vi "Handle Command.vi"(8 "error in (no error)":errorcluster, 9 "Data":variant, 10 "Command":string, 11 "Inst.Xeryon-Rotator in":refnum<class "Inst.Xeryon-Rotator.lvclass">) -> (0 "error out":errorcluster, 1 "Processed Data":variant, 2 "Command":string, 3 "Inst.Xeryon-Rotator out":refnum<class "Inst.Xeryon-Rotator.lvclass">)   [LabVIEW 2019, in "Inst.Xeryon-Rotator.lvclass"]
uses:
  Inst.Xeryon-Rotator.lvclass
  Inst.Xeryon-Rotator.lvclass/Inst.Xeryon-Rotator.ctl
  <userlib>/LevyLab/Instrument Framework/Instrument Types/Cryostat/Instrument.Cryostat.lvclass
  <userlib>/LevyLab/Instrument Framework/Instrument Types/Cryostat/Typedefs/getAngle--cluster.ctl
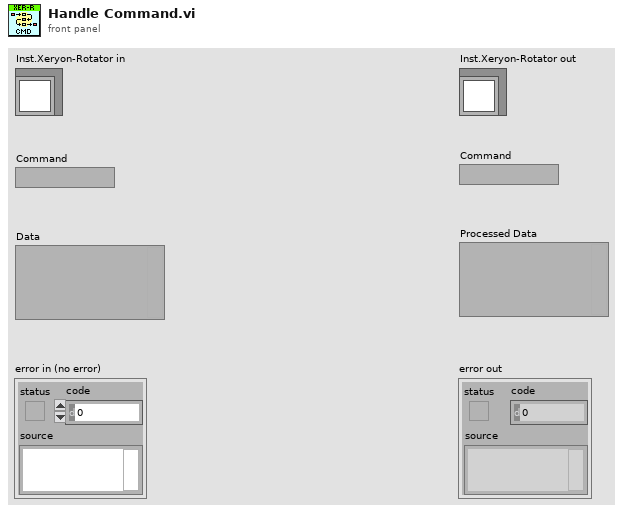
[diagram p1: front panel]
types:
  T1 = typedef "Instrument.Cryostat.lvclass/getAngle--cluster.ctl" = cluster{"angle":dbl, "status":string, "finished":bool}
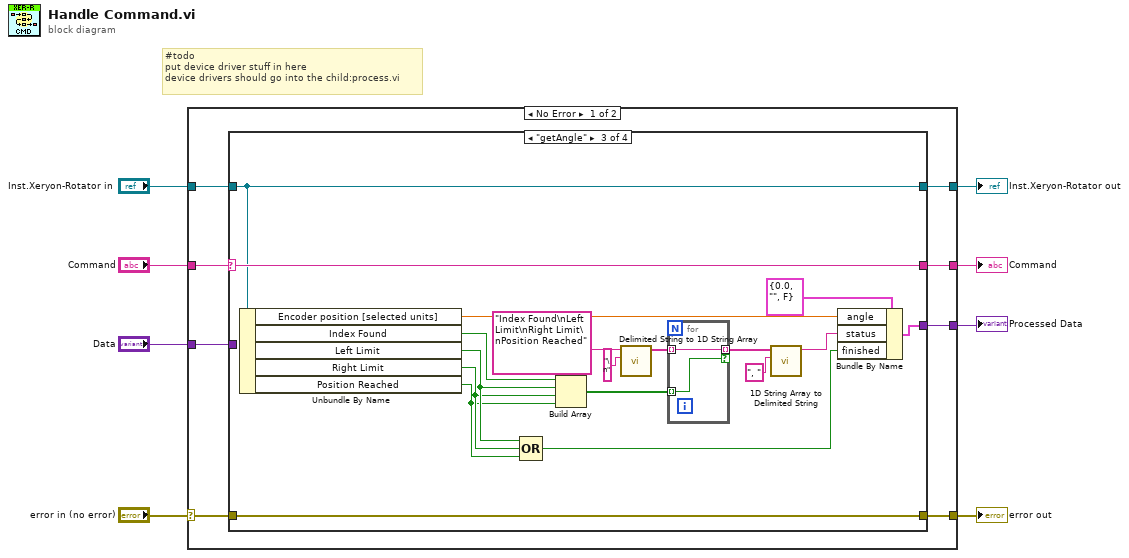
[diagram p0: block diagram]
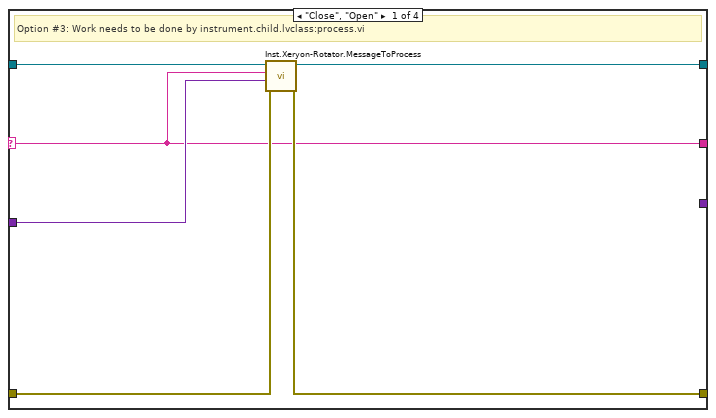
[diagram p2: hidden frame]
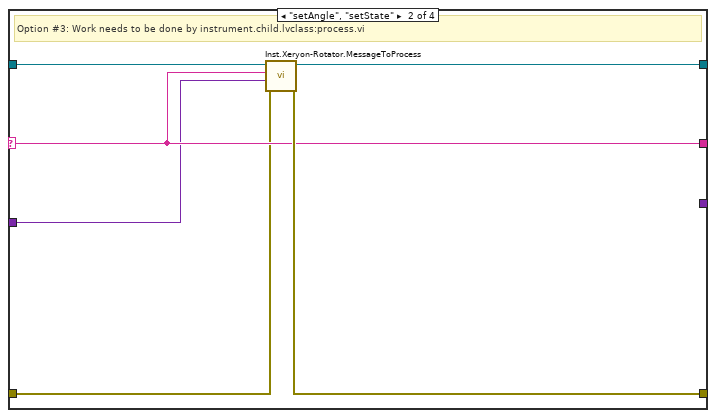
[diagram p3: hidden frame]
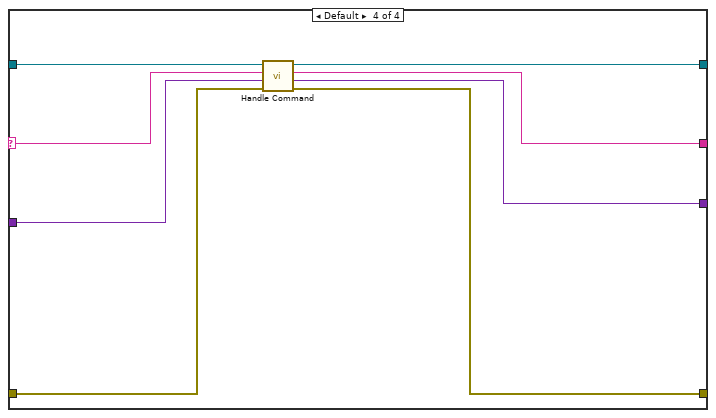
[diagram p4: hidden frame]
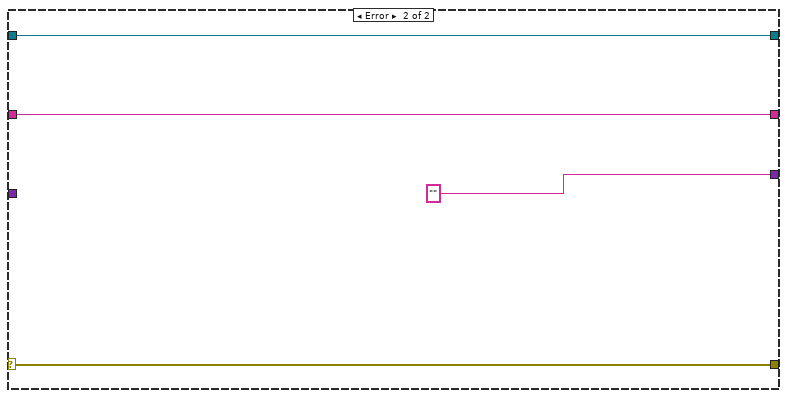
[diagram p5: hidden frame]
diagram:
  # "#todo\nput device driver stuff in here\ndevice drivers should go into the child:process.vi"
  n1 = case shown="No Error" "error in (no error)" {
    selector: "error in (no error)" -> [w10 w60]
    tunnel: [w12 w60] -> w6
    tunnel: [w14 w59] -> w5
    tunnel: "Inst.Xeryon-Rotator in" -> [w15 w59]
    tunnel: "Command" -> [w16 w57]
    tunnel: [w13 "" ("String")] -> w3
    tunnel: "Data" -> [w9 _]
    tunnel: [w11 w57] -> w1
    frame No Error {
      n2 = case shown="\"getAngle\"" w16 {
        selector: w16 -> [w17 w25 w46 w50]
        tunnel: w15 -> [w22 w28 w45 w54]
        tunnel: [w21 w27 w45 w51] -> w14
        tunnel: [_ _ w41 w53] -> w13
        tunnel: w10 -> [w20 w23 w42 w55]
        tunnel: w9 -> [w18 w24 _ w56]
        tunnel: [w19 w26 w42 w52] -> w12
        tunnel: [w17 w25 w46 w49] -> w11
        frame "Close", "Open" {
          # "Option #3: Work needs to be done by instrument.child.lvclass:process.vi"
          n3 = call "Inst.Xeryon-Rotator.MessageToProcess.vi"("error in (no error)"=w20, "Data"=w18, "Command"=w17, "Inst.Xeryon-Rotator in"=w22) -> ("error out"=w19:errorcluster, "Inst.Xeryon-Rotator out"=w21:refnum<class "Inst.Xeryon-Rotator.lvclass">)  [unwired: 6 in]
        }
        frame "setAngle", "setState" {
          # "Option #3: Work needs to be done by instrument.child.lvclass:process.vi"
          n4 = call "Inst.Xeryon-Rotator.MessageToProcess.vi"("error in (no error)"=w23, "Data"=w24, "Command"=w25, "Inst.Xeryon-Rotator in"=w28) -> ("error out"=w26:errorcluster, "Inst.Xeryon-Rotator out"=w27:refnum<class "Inst.Xeryon-Rotator.lvclass">)  [unwired: 6 in]
        }
        frame "getAngle" {
          n5 = Unbundle By Name(w45) -> ("Encoder position [selected units]"=w43:dbl, "Index Found"=w37:bool, "Left Limit"=w32:bool, "Right Limit"=w31:bool, "Position Reached"=w30:bool)
          n6 = Compound Arithmetic op=OR(w32, w31, w30) -> (w29:bool)
          n7 = Build Array(w37, w32, w31, w30) -> (w33:bool[])
          n8 = call <vilib>:"Delimited String to 1D String Array.vi"("delimiter"="\n", "delimited string"="Index Found\nLeft Limit\nRight Limit\nPosition Reached") -> ("string array"=w36:string[])  [unwired: 9 in]
          n9 = for {
            tunnel: [w48] -> w34 mode=indexing if=w47
            tunnel: w36 -> [w48] mode=indexing
            tunnel: w33 -> [w47] mode=indexing
          }
          n10 = call <vilib>:"1D String Array to Delimited String.vi"("delimiter"=", ", "string array"=w34) -> ("delimited string"=w40:string)  [unwired: 9 in]
          n11 = Bundle By Name(cluster=T1 {"angle"=0.0, "status"="", "finished"=FALSE} ("getAngle"), "angle"=w43, "status"=w40, "finished"=w29) -> (w41:T1)
        }
        frame Default {
          n12 = call-parent "Handle Command.vi"("error in (no error)"=w55, "params in"=w56, "command"=w50, "Instrument in"=w54) -> ("error out"=w52:errorcluster, "processed data"=w53:variant, "command out"=w49:string, "Instrument out"=w51:refnum<class "Inst.Xeryon-Rotator.lvclass">)  [unwired: 4 in]
        }
      }
    }
    frame Error {
    }
  }
  "error out" <- w6
  "Inst.Xeryon-Rotator out" <- w5
  "Command" <- w1
  "Processed Data" <- w3
